vi "期末.vi"() -> ()   [LabVIEW 2014]
panel:
  in  "粗體":bool
  in  "底線":bool
  in  "斜體":bool
  in  "跑馬燈速度":i32(knob) caption="Knob" scale=50.0..200.0
  in  "String":string
  in  "stop":bool
  in  "暫停":bool
  in  "Enter":bool
  out "LED panel":bool[][](array[boolean])
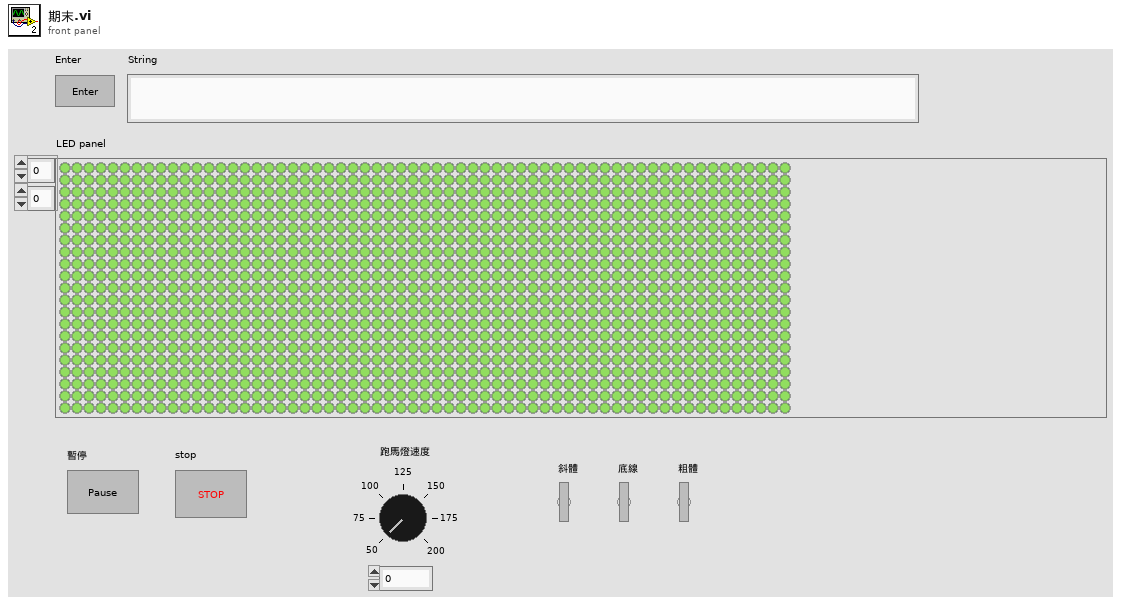
[diagram p1: front panel]
types:
  T1 = cluster{"left":i16, "top":i16, "right":i16, "bottom":i16}
  T2 = enum16{"User-specified Font", "Application Font", "System Font", "Dialog Font"}
  T3 = cluster{"Font Name:":string, "Size":i16, "Strikeout?":bool, "Italic?":bool, "Underline?":bool, "Outline?":bool, "Shadow?":bool, "Bold?":bool}
  T4 = typedef "imagedata.ctl" = cluster{"image type":i32, "image depth":i32, "image":u8[], "mask":u8[], "colors":u32[], "Rectangle":cluster{"left":i16, "top":i16, "right":i16, "bottom":i16}}
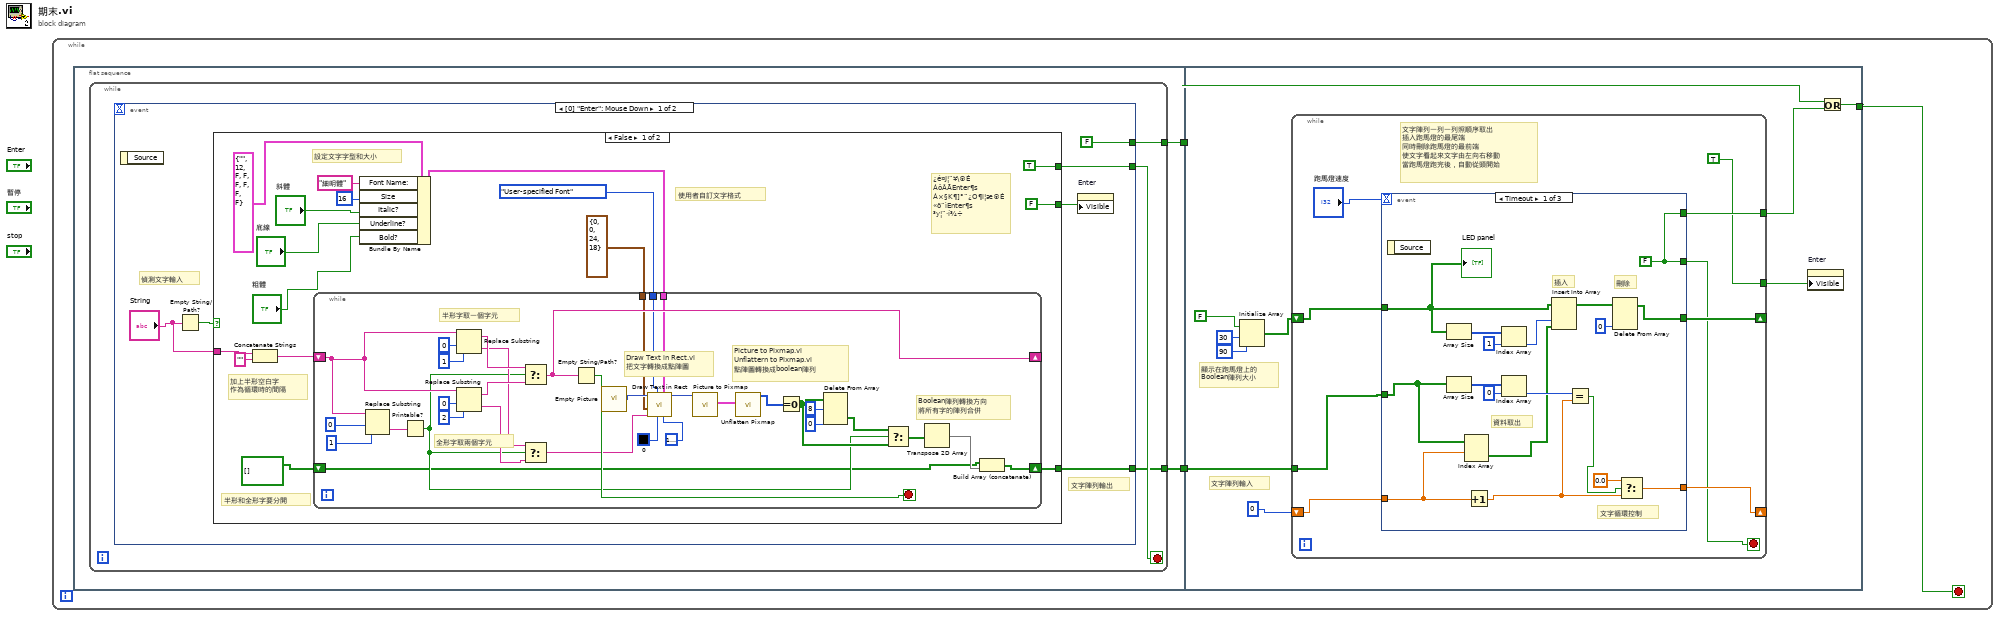
[diagram p0: block diagram]
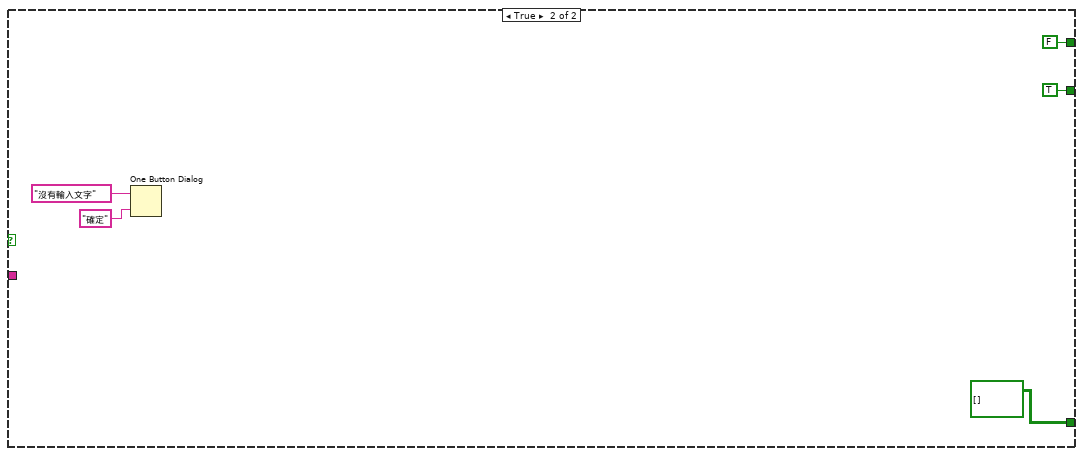
[diagram p2: hidden frame]
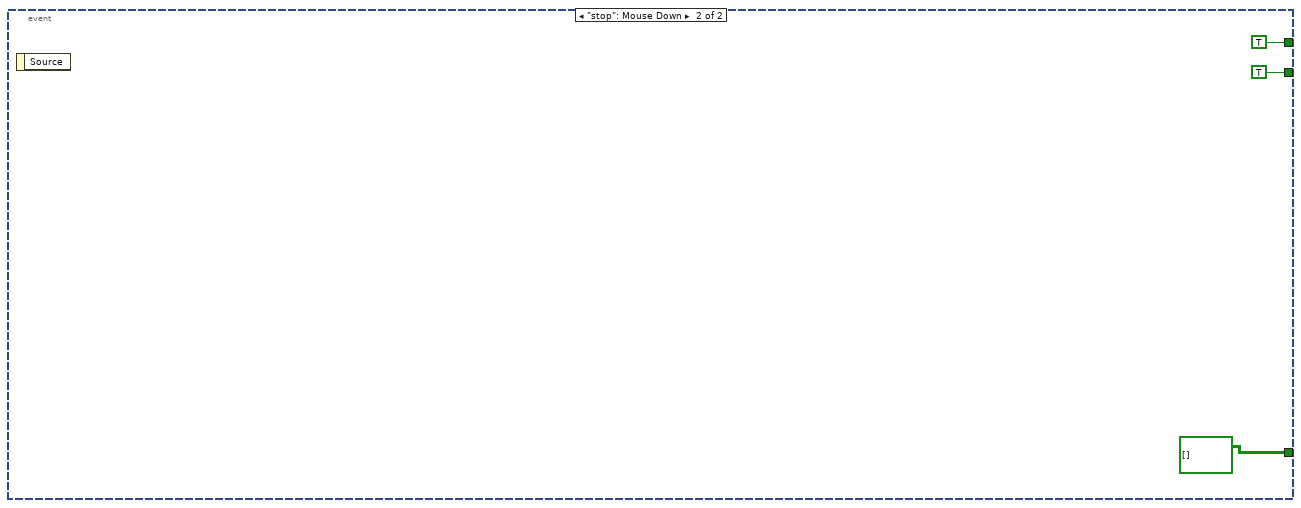
[diagram p3: hidden frame]
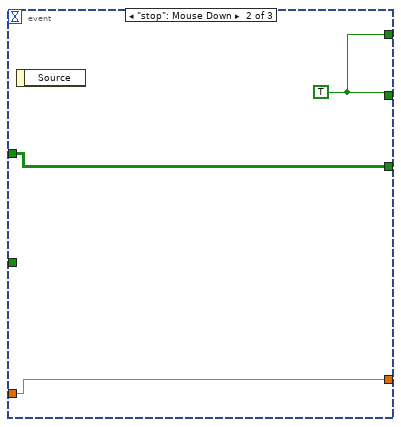
[diagram p4: hidden frame]
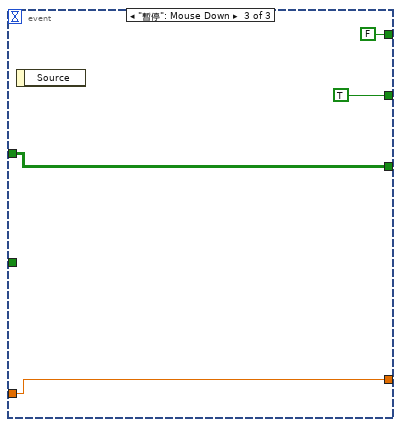
[diagram p5: hidden frame]
diagram:
  n1 = while {
    stop <- w1 stop-if-true
    n2 = flat-sequence {
      tunnel: [w5] -> w3
      tunnel: [w4] -> w2
      tunnel: w3 -> [w81]
      tunnel: w2 -> [w75]
      tunnel: [w80] -> w1
      frame #0 {
        n3 = while {
          tunnel: [w7] -> w5
          tunnel: [w6] -> w4
          stop <- w8 stop-if-true
          n4 = event shown="[0] \"Enter\": Mouse Down" {
            selector: _ -> [_ _]
            dyn-events: _ -> [_ _]
            timeout: _ -> [_ _]
            tunnel: [w11 TRUE] -> w8
            tunnel: [FALSE TRUE] -> w7
            tunnel: [w9 bool[][] []] -> w6
            event "Enter": Mouse Down {
              # "文字陣列輸出"
              # "偵測文字輸入"
              n5 = event-data() -> ()  [unwired: 1 in, 1 out]
              n6 = Empty String/Path?(string/path="String") -> (empty?=w14:bool)
              n7 = case shown="False" w14 {
                tunnel: "String" -> [w30 _]
                tunnel: [FALSE TRUE] -> w12
                tunnel: [TRUE FALSE] -> w11
                tunnel: [w18 bool[][] []] -> w9
                frame False {
                  # "¿é¤J¦¨¥\\®É\nÁôÂÃEnter¶s\nÁ×§K¶]°¨¿O¶i¦æ®É\n«ö¨ìEnter¶s\n³y¦¨·í¾÷"
                  # "使用者自訂文字格式"
                  # "半形和全形字要分開"
                  # "加上半形空白字\n作為循環時的間隔"
                  # "設定文字字型和大小"
                  n8 = Concatenate Strings(w30, "" ("string")) -> (w28:string)
                  n9 = Bundle By Name(cluster=T3 {"Font Name:"="", "Size"=12, "Strikeout?"=FALSE, "Italic?"=FALSE, "Underline?"=FALSE, "Outline?"=FALSE, "Shadow?"=FALSE, "Bold?"=FALSE} ("[user-specified font]"), "Font Name:"="細明體", "Size"=i16 16, "Italic?"="斜體", "Underline?"="底線", "Bold?"="粗體") -> (w23:T3)
                  n10 = while {
                    shift-right: [w51] -> _
                    shift-left: w28 -> [w60]
                    shift-right: [w36] -> w18
                    shift-left: bool[][] [] -> [w31]
                    tunnel: w23 -> [w35]
                    tunnel: T2."User-specified Font" ("desired font(Application)") -> [w34]
                    tunnel: T1 {"left"=0, "top"=0, "right"=24, "bottom"=18} ("rect") -> [w33]
                    stop <- w50 stop-if-true
                    # "Boolean陣列轉換方向\n將所有字的陣列合併"
                    # "Picture to Pixmap.vi\nUnflattern to Pixmap.vi\n點陣圖轉換成boolean陣列"
                    # "Draw Text in Rect.vi\n把文字轉換成點陣圖"
                    # "全形字取兩個字元"
                    # "半形字取一個字元"
                    n11 = Replace Substring(2:1 ("length (len. of substring)"), 3:0 ("offset (0)"), 5:w60) -> (0:w61:string)  [unwired: 1 in, 1 out]
                    n12 = Printable?(1:w61) -> (0:w38:bool)
                    n13 = Replace Substring(2:1 ("length (len. of substring)"), 3:0 ("offset (0)"), 5:w60) -> (0:w53:string, 1:w55:string)  [unwired: 1 in]
                    n14 = Replace Substring(2:2 ("length (len. of substring)"), 3:0 ("offset (0)"), 5:w60) -> (0:w52:string, 1:w54:string)  [unwired: 1 in]
                    n15 = Select(t=w55, s=w38, f=w54) -> (s? t:f=w51:string)
                    n16 = Select(t=w53, s=w38, f=w52) -> (s? t:f=w49:string)
                    n17 = Empty String/Path?(string/path=w51) -> (empty?=w50:bool)
                    n18 = call "Empty Picture"() -> ("empty picture"=w48:picture)
                    n19 = call <vilib>:"Draw Text in Rect.vi"("BG color(transparent)"=u32 16777226, "[user-specified font]"=w35, "text color(black)"=u32 0, "desired font(Application)"=w34, "text"=w49, "rect"=w33, "picture"=w48) -> ("new picture"=w47:picture)  [unwired: 4 in]
                    n20 = call <vilib>:"Picture to Pixmap.vi"("picture"=w47) -> ("image data"=w46:T4)  [unwired: 9 in, 1 out]
                    n21 = call <vilib>:"Unflatten Pixmap.vi"("image data"=w46) -> ("24-bit pixmap"=w45:u32[][])  [unwired: 4 in, 6 out]
                    n22 = Equal To 0?(x=w45) -> (x = 0?=w39:bool[][])
                    n23 = Delete From Array(array=w39, length=8, index (col)=0 ("disabled index (col)")) -> (deleted portion=w40:bool[][])  [unwired: 1 in, 1 out]
                    n24 = Select(t=w40, s=w38, f=w39) -> (s? t:f=w37:bool[][])
                    n25 = Transpose 2D Array(2D array=w37) -> (transposed array=w32:bool[][])
                    n26 = Build Array (concatenate)(w31, w32) -> (w36:bool[][])
                  }
                }
                frame True {
                  n27 = One Button Dialog(message="沒有輸入文字", button name ("OK")="確定") -> ()  [unwired: 1 out]
                }
              }
              n28 = property on="Enter" class="Bool"("Visible"=w12) -> ()  [unwired: 2 in, 2 out]
            }
            event "stop": Mouse Down {
              n29 = event-data() -> ()  [unwired: 1 in, 1 out]
            }
          }
        }
      }
      frame #1 {
        # "文字陣列輸入"
        # "顯示在跑馬燈上的\nBoolean陣列大小"
        n30 = Initialize Array(FALSE, 30 ("dimension size"), 90 ("dimension size")) -> (w76:bool[][])
        n31 = while {
          shift-right: [w87] -> _
          shift-left: w76 -> [w89]
          tunnel: w75 -> [w88]
          shift-right: [w85] -> _
          shift-left: 0 -> [w86]
          tunnel: [w83] -> w73
          tunnel: [TRUE] -> w72
          stop <- w84 stop-if-true
          # "文字陣列一列一列照順序取出\n插入跑馬燈的最尾端\n同時刪除跑馬燈的最前端\n使文字看起來文字由左向右移動\n當跑馬燈跑完後，自動從頭開始"
          n32 = event shown="[0] Timeout" {
            selector: _ -> [_ _ _]
            dyn-events: _ -> [_ _ _]
            timeout: "跑馬燈速度" -> [_ _ _]
            tunnel: w89 -> [w91 w111 w115]
            tunnel: w88 -> [w99 _ _]
            tunnel: [w101 w111 w115] -> w87
            tunnel: w86 -> [w98 w109 w112]
            tunnel: [w93 w109 w112] -> w85
            tunnel: [w92 w110 TRUE] -> w84
            tunnel: [w92 w110 FALSE] -> w83
            event Timeout {
              w92 = FALSE
              # "文字循環控制"
              # "刪除"
              # "插入"
              # "資料取出"
              n33 = event-data() -> ()  [unwired: 1 in, 1 out]
              n34 = Array Size(array=w91) -> (size(s)=w108:i32[])
              n35 = Array Size(array=w99) -> (size(s)=w106:i32[])
              n36 = Index Array(array=w99, index (row)=w98) -> (element=w97:bool[])  [unwired: 1 in]
              n37 = Increment(x=w98) -> (x+1=w95:dbl)
              n38 = Index Array(array=w108, index=1) -> (element=w104:i32)
              n39 = Index Array(array=w106, index=0) -> (element=w100:i32)
              n40 = Insert Into Array(array=w91, index (col)=w104, new element=w97) -> (w102:bool[][])  [unwired: 1 in]
              n41 = Equal?(x=w100, y=w95) -> (x = y?=w94:bool)
              n42 = Delete From Array(array=w102, index (col)=0) -> (array with subset deleted=w101:bool[][])  [unwired: 2 in, 1 out]
              n43 = Select(t=0.0, s=w94, f=w95) -> (s? t:f=w93:dbl)
              "LED panel" <- w91
            }
            event "stop": Mouse Down {
              w110 = TRUE
              n44 = event-data() -> ()  [unwired: 1 in, 1 out]
            }
            event "暫停": Mouse Down {
              n45 = event-data() -> ()  [unwired: 1 in, 1 out]
            }
          }
        }
        n46 = property on="Enter" class="Bool"("Visible"=w72) -> ()  [unwired: 2 in, 2 out]
        n47 = Or(x=w81, y=w73) -> (x .or. y?=w80:bool)
      }
    }
  }
